vi "scene_object with scale and shift.vi"(8 "error in (no error)":errorcluster, 9 "scale":sgl=1.0, 10 "point3f - SHIFT":T2 {"z" format="%.2f"; "y" format="%.2f"; "x" format="%.2f"}, 11 "Object In":T1 {"NormalList"."z" format="%.2f"; "NormalList"."y" format="%.2f"; "NormalList"."x" format="%.2f"; "VertexList"."z" format="%.2f"; "VertexList"."y" format="%.2f"; "VertexList"."x" format="%.2f"}) -> (0 "error out":errorcluster, 3 "SceneMesh out":refnum<vi>, 4 "Object Out":T1={"VertexList"=[], "FaceList"=[], "NormalList"=[], "Mode"=enum."GL_TRIANGLES"} {"NormalList"."z" format="%.2f"; "NormalList"."y" format="%.2f"; "NormalList"."x" format="%.2f"; "VertexList"."z" format="%.2f"; "VertexList"."y" format="%.2f"; "VertexList"."x" format="%.2f"}, 5 "FaceList":cluster{"v1":i32, "v2":i32, "v3":i32}[](array[cluster]), 7 "Array":T2[](array[typedef]) {"z" format="%.2f"; "y" format="%.2f"; "x" format="%.2f"})   [LabVIEW 2026, in "3D utilities.lvlib"]
uses:
  3D utilities.lvlib
  <vilib>/picture/3D Picture Control/Old 3D Toolkit.llb/model.ctl
  <vilib>/picture/3D Picture Control/Old 3D Toolkit.llb/point3f.ctl
  <vilib>/picture/3D Picture Control/Old 3D Toolkit.llb/VertexMode.ctl
  <vilib>/picture/3D Picture Control/NI_Old 3D Toolkit.lvlib
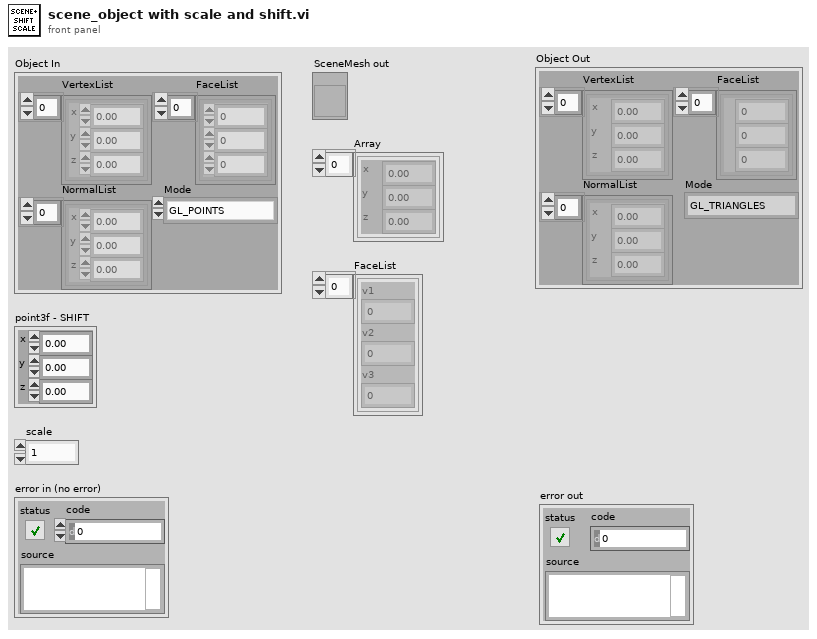
[diagram p1: front panel]
types:
  T1 = typedef "NI_3D Picture Control.lvlib/NI_Old 3D Toolkit.lvlib/model.ctl" = cluster{"VertexList":T2[], "FaceList":cluster{"v1":i32, "v2":i32, "v3":i32}[], "NormalList":T2[], "Mode":T3}
  T2 = typedef "NI_3D Picture Control.lvlib/NI_Old 3D Toolkit.lvlib/point3f.ctl" = cluster{"x":sgl, "y":sgl, "z":sgl}
  T3 = typedef "NI_3D Picture Control.lvlib/NI_Old 3D Toolkit.lvlib/VertexMode.ctl" = enum16{"GL_POINTS", "GL_LINES", "GL_LINE_LOOP", "GL_LINE_STRIP", "GL_TRIANGLES", "GL_TRIANGLE_STRIP", "GL_TRIANGLE_FAN", "GL_QUADS", "GL_QUAD_STRIP", "GL_POLYGON"}
  T4 = enum16{"Overall", "Per Primitive", "Per Vertex", "Binding Off"}
  T5 = enum16{"Points", "Lines", "Line Strip", "Line Loop", "Triangles", "Triangle Strip", "Triangle Fan", "Quads", "Quad Strip", "Polygon"}
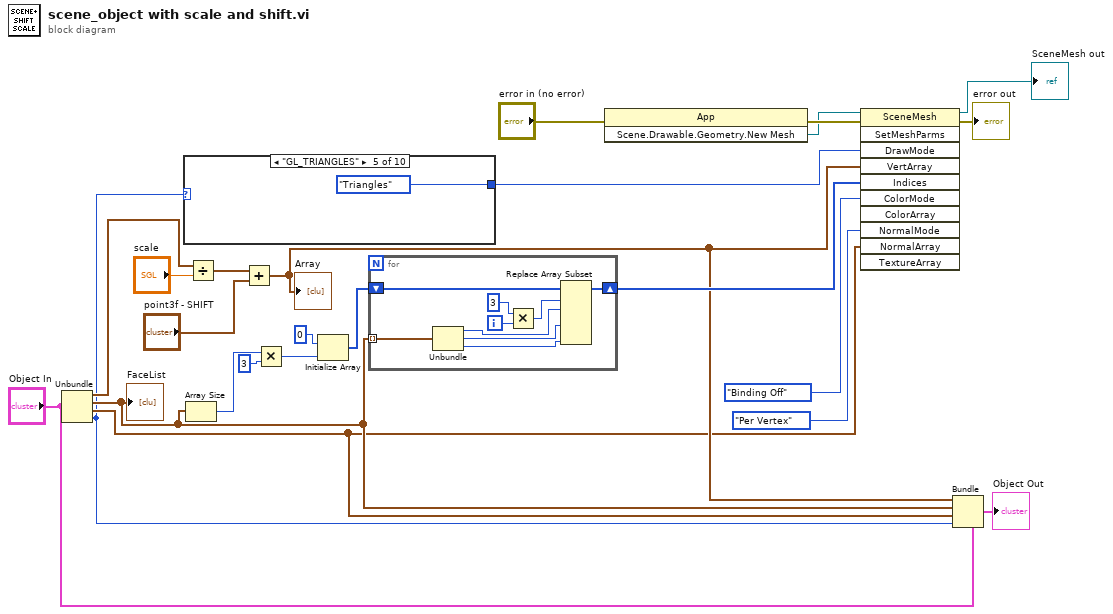
[diagram p0: block diagram]
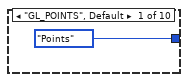
[diagram p2: hidden frame]
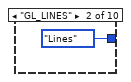
[diagram p3: hidden frame]
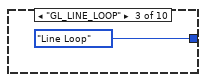
[diagram p4: hidden frame]
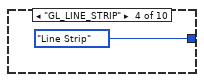
[diagram p5: hidden frame]
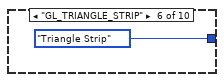
[diagram p6: hidden frame]
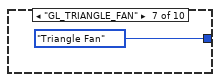
[diagram p7: hidden frame]
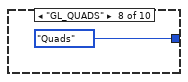
[diagram p8: hidden frame]
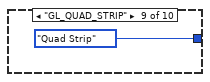
[diagram p9: hidden frame]
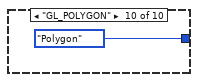
[diagram p10: hidden frame]
diagram:
  n1 = Unbundle("Object In") -> ("VertexList"=w23:T2[], "FaceList"=w4:cluster{"v1":i32, "v2":i32, "v3":i32}[], "NormalList"=w3:T2[], "Mode"=w2:T3)
  "FaceList" <- w4
  n2 = case shown="\"GL_TRIANGLES\"" w2 {
    tunnel: [T5."Points" ("Draw Mode") T5."Lines" ("Draw Mode") T5."Line Loop" ("Draw Mode") T5."Line Strip" ("Draw Mode") T5."Triangles" ("Draw Mode") T5."Triangle Strip" ("Draw Mode") T5."Triangle Fan" ("Draw Mode") T5."Quads" ("Draw Mode") T5."Quad Strip" ("Draw Mode") T5."Polygon" ("Draw Mode")] -> w11
    frame "GL_POINTS", Default {
    }
    frame "GL_LINES" {
    }
    frame "GL_LINE_LOOP" {
    }
    frame "GL_LINE_STRIP" {
    }
    frame "GL_TRIANGLES" {
    }
    frame "GL_TRIANGLE_STRIP" {
    }
    frame "GL_TRIANGLE_FAN" {
    }
    frame "GL_QUADS" {
    }
    frame "GL_QUAD_STRIP" {
    }
    frame "GL_POLYGON" {
    }
  }
  n3 = Array Size(array=w4) -> (size(s)=w15:i32)
  n4 = Divide(x=w23, y="scale") -> (x/y=w24:T2[])
  n5 = Add(x=w24, y="point3f - SHIFT") -> (x+y=w5:T2[])
  "Array" <- w5
  n6 = Multiply(x=w15, y=3 ("x")) -> (x*y=w16:i32)
  n7 = Initialize Array(0 ("v3"), w16) -> (w12:i32[])
  n8 = for {
    tunnel: w4 -> [w43] mode=indexing
    shift-right: [w42] -> w10
    shift-left: w12 -> [w41]
    i -> [w37]
    n9 = Unbundle(w43) -> ("v1"=w40:i32, "v2"=w39:i32, "v3"=w38:i32)
    n10 = Multiply(x=3, y=w37) -> (x*y=w35:i32)
    n11 = Replace Array Subset(array=w41, new element #1=w40, index #1=w35, new element #2=w39, new element #3=w38) -> (w42:i32[])  [unwired: 2 in]
  }
  n12 = invoke class="App" method="Scene.Drawable.Geometry.New Mesh"(error in="error in (no error)") -> (error out=w8:errorcluster, "Scene.Geometry.New Mesh"=w7:refnum<vi>)  [unwired: 2 in, 1 out]
  n13 = invoke class="SceneMesh" method="SetMeshParms"(reference=w7, error in=w8, "DrawMode"=w11, "VertArray"=w5, "Indices"=w10, "ColorMode"=T4."Binding Off" ("Color Binding Mode"), "NormalMode"=enum16{"Overall", "Per Primitive", "Per Vertex"}."Per Vertex" ("Normal Binding Mode"), "NormalArray"=w3) -> (reference out=→"SceneMesh out":refnum<vi>, error out=→"error out":errorcluster)  [unwired: 3 in, 9 out]
  n14 = Bundle(cluster="Object In", "VertexList"=w5, "FaceList"=w4, "NormalList"=w3, "Mode"=w2) -> (→"Object Out":T1)
